vi "set background and target(normal mode).vi"(8 "number of targets":i32=10, 10 "spacing limit":i32=30, 11 "new picture":picture) -> (0 "Array 2":cluster{"Numeric":i32, "Numeric 2":i32}[](array[cluster]), 2 "new picture 3":picture)   [LabVIEW 2014]
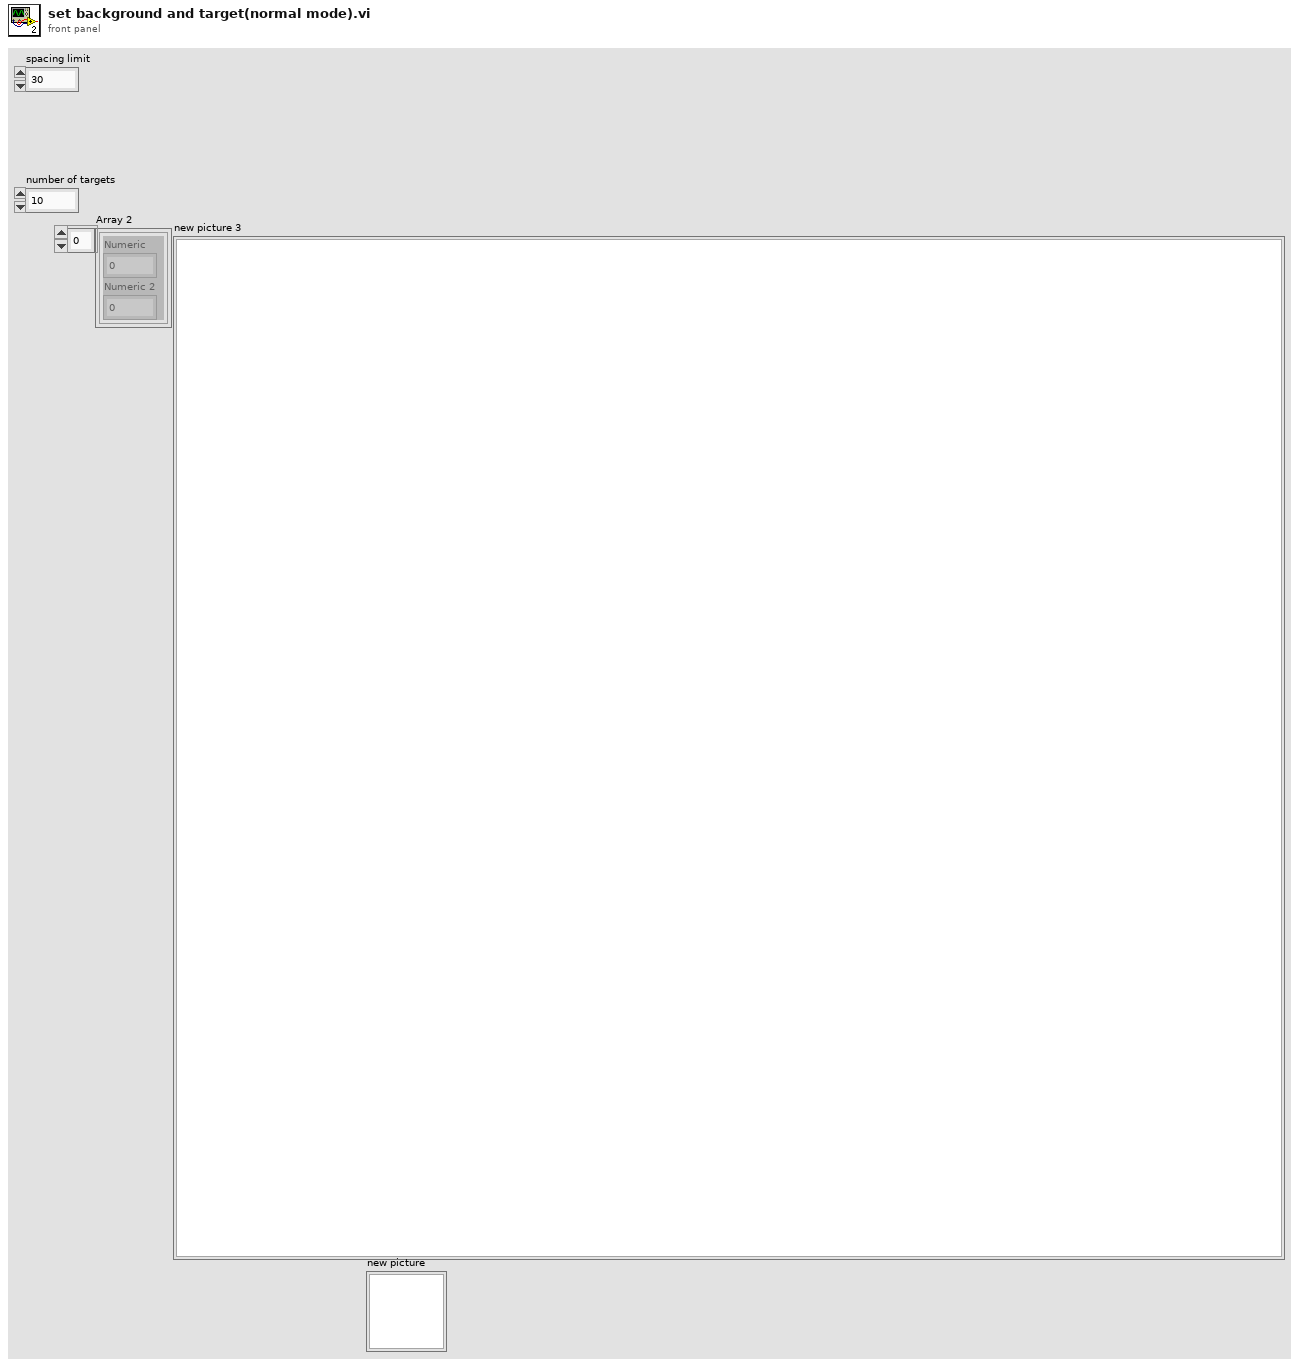
[diagram p1: front panel]
types:
  T1 = typedef "LVBoundsTypeDef.ctl" = cluster{"Width":u32, "Height":u32}
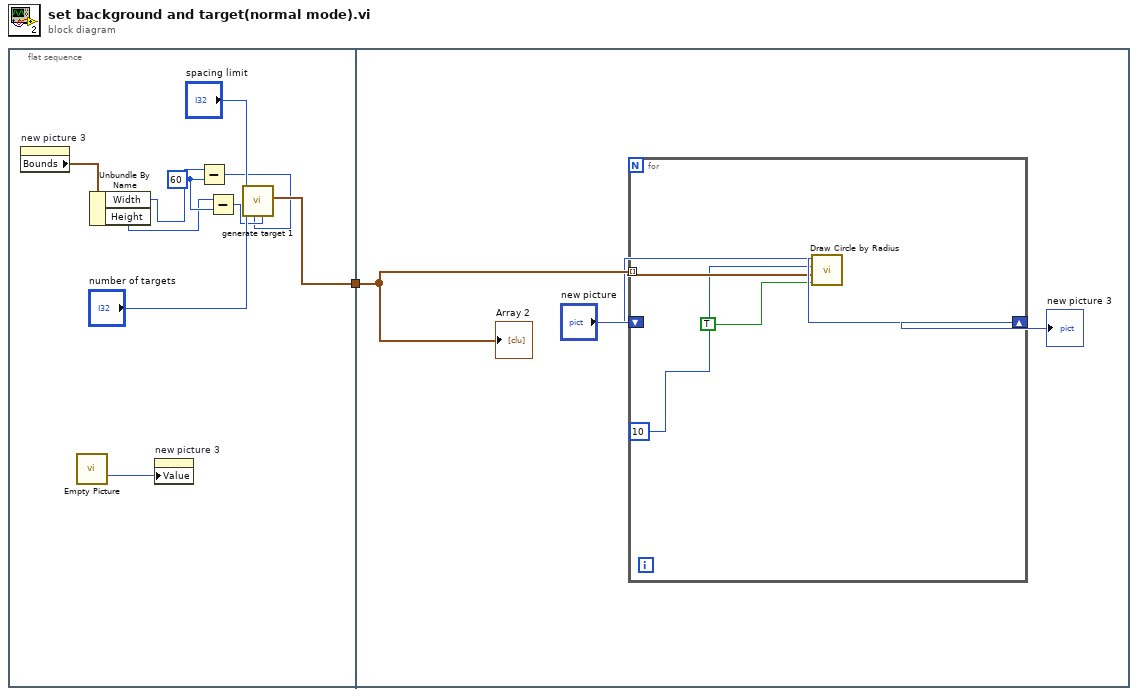
[diagram p0: block diagram]
diagram:
  n1 = flat-sequence {
    tunnel: [w10] -> w1
    tunnel: w1 -> [w13]
    frame #0 {
      w6 = u32 60 ("y")
      n2 = property on="new picture 3" class="Pict"() -> ("Bounds"=w11:T1)  [unwired: 2 in, 2 out]
      n3 = call "Empty Picture"() -> ("empty picture"=w2:picture)
      n4 = Unbundle By Name(w11) -> ("Width"=w7:u32, "Height"=w5:u32)
      n5 = property on="new picture 3" class="Pict"("Value"=w2) -> ()  [unwired: 2 in, 2 out]
      n6 = Subtract(x=w7, y=w6) -> (x-y=w3:u32)
      n7 = Subtract(x=w5, y=w6) -> (x-y=w4:u32)
      n8 = call "generate target 1.vi"("PICTURE SIZE Y"=w4, "PICTURE SIZE X"=w3, "number of targets"="number of targets", "spacing limit"="spacing limit") -> ("Array 2"=w10:cluster{"Numeric":i32, "Numeric 2":i32}[])  [unwired: 7 in]
    }
    frame #1 {
      n9 = for {
        shift-right: [w19] -> w14
        shift-left: "new picture" -> [w15]
        tunnel: w13 -> [w18] mode=indexing
        n10 = call <vilib>:"Draw Circle by Radius.vi"("fill?(F)"=TRUE, "pixel center"=w18, "radius"=i16 10, "picture"=w15) -> ("new picture"=w19:picture)  [unwired: 7 in]
      }
      "new picture 3" <- w14
      "Array 2" <- w13
    }
  }
